vi "Global_SM_Data Out.vi"() -> ()   [LabVIEW 2017, in "TemplateActuator.lvlib"]
uses:
  TemplateActuator.lvlib
  Cluster_SM To HW Data.ctl
  Cluster_SM Status.ctl
panel:
  in  "SM_Actuator_Status":T1
  in  "SM_Actuator_HW Data":T2
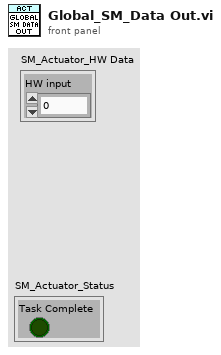
[diagram p1: front panel]
types:
  T1 = typedef "TemplateActuator.lvlib/Cluster_SM Status.ctl" = cluster{"Task Complete":bool}
  T2 = typedef "TemplateActuator.lvlib/Cluster_SM To HW Data.ctl" = cluster{"HW input":dbl}
diagram:
